vi "Resize FP.vi"(0 "VI in":refnum<vi>, 11 "error in":errorcluster) -> (4 "VI out":refnum<vi>, 15 "error out":errorcluster)   [LabVIEW 2017, in "Align To Connector.lvlib"]
uses:
  Align To Connector.lvlib
  <vilib>/Utility/miscctls.llb/LVRectTypeDef.ctl
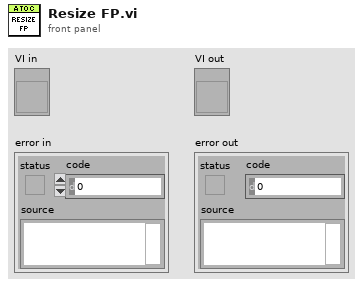
[diagram p1: front panel]
types:
  T1 = typedef "LVRectTypeDef.ctl" = cluster{"Left":i16, "Top":i16, "Right":i16, "Bottom":i16}
  T2 = typedef "LVPointTypeDef.ctl" = cluster{"Horizontal":i16, "Vertical":i16}
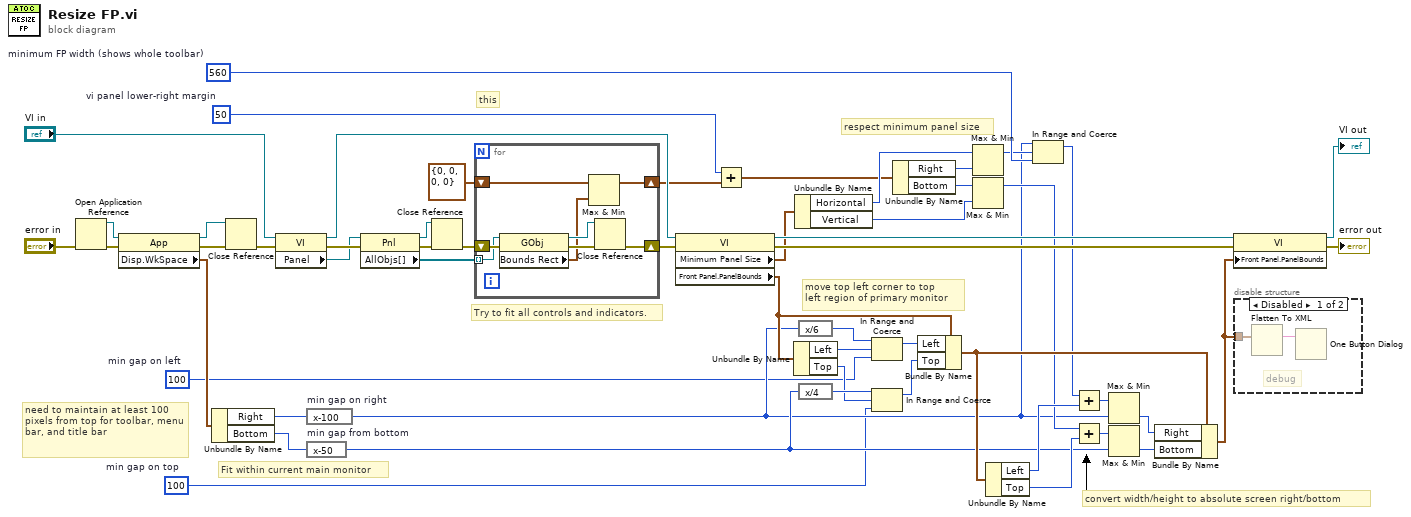
[diagram p0: block diagram]
diagram:
  w1 = i16 50  # vi panel lower-right margin
  w4 = i16 100  # min gap on left
  w7 = i16 100  # min gap on top
  w21 = i16 560  # minimum FP width (shows whole toolbar)
  # "this"
  # "respect minimum panel size"
  # "need to maintain at least 100 pixels from top for toolbar, menu bar, and title bar"
  # "move top left corner to top\nleft region of primary monitor"
  # "convert width/height to absolute screen right/bottom"
  # "Try to fit all controls and indicators."
  # "Fit within current main monitor"
  n1 = Open Application Reference(8:"error in") -> (0:w42:errorcluster, 3:w45:refnum<vi>)  [unwired: 3 in]
  n2 = property class="App"(reference=w45, error in=w42) -> (reference out=w44:refnum<vi>, error out=w43:errorcluster, "Disp.WkSpace"=w15:T1)
  n3 = Unbundle By Name(w15) -> ("Right"=w39:i16, "Bottom"=w38:i16)
  n4 = Close Reference(reference=w44, error in (no error)=w43) -> (error out=w40:errorcluster)
  n5 = property class="VI"(reference="VI in", error in=w40) -> (reference out=w30:refnum<vi>, error out=w35:errorcluster, "Panel"=w31:refnum<vi>)
  n6 = expression code="x-100" "min gap on right"(w39) -> (w10:i16)
  n7 = expression code="x-50" "min gap from bottom"(w38) -> (w20:i16)
  n8 = property class="Pnl"(reference=w31, error in=w35) -> (reference out=w33:refnum<vi>, error out=w34:errorcluster, "AllObjs[]"=w36:refnum<vi>[])
  n9 = Close Reference(reference=w33, error in (no error)=w34) -> (error out=w51:errorcluster)
  n10 = for {
    tunnel: w36 -> [w55] mode=indexing
    shift-right: [w60] -> w32
    shift-left: w51 -> [w62]
    shift-right: [w56] -> w11
    shift-left: T1 {"Left"=0, "Top"=0, "Right"=0, "Bottom"=0} ("Bounds Rect") -> [w57]
    n11 = property class="GObj"(reference=w55, error in=w62) -> (reference out=w59:refnum<vi>, error out=w61:errorcluster, "Bounds Rect"=w58:T1)
    n12 = Max & Min(x=w57, y=w58) -> (max(x,y)=w56:T1)  [unwired: 1 out]
    n13 = Close Reference(reference=w59, error in (no error)=w61) -> (error out=w60:errorcluster)
  }
  n14 = property class="VI"(reference=w30, error in=w32) -> (reference out=w52:refnum<vi>, error out=w50:errorcluster, "Minimum Panel Size"=w5:T2, "Front Panel.PanelBounds"=w16:T1)
  n15 = Add(x=w1, y=w11) -> (x+y=w2:T1)
  n16 = Unbundle By Name(w16) -> ("Left"=w53:i16, "Top"=w8:i16)
  n17 = Unbundle By Name(w5) -> ("Horizontal"=w14:i16, "Vertical"=w3:i16)
  n18 = expression code="x/6"(w10) -> (w19:i16)
  n19 = expression code="x/4"(w20) -> (w9:i16)
  n20 = In Range and Coerce(upper limit=w19, x=w53, lower limit=w4) -> (coerced(x)=w18:i16)  [unwired: 1 out]
  n21 = In Range and Coerce(upper limit=w9, x=w8, lower limit=w7) -> (coerced(x)=w17:i16)  [unwired: 1 out]
  n22 = Unbundle By Name(w2) -> ("Right"=w28:i16, "Bottom"=w27:i16)
  n23 = Bundle By Name(cluster=w16, "Left"=w18, "Top"=w17) -> (w54:T1)
  n24 = Max & Min(x=w14, y=w28) -> (max(x,y)=w13:i16)  [unwired: 1 out]
  n25 = Max & Min(x=w27, y=w3) -> (max(x,y)=w12:i16)  [unwired: 1 out]
  n26 = Unbundle By Name(w54) -> ("Left"=w46:i16, "Top"=w37:i16)
  n27 = In Range and Coerce(upper limit=w10, x=w13, lower limit=w21) -> (coerced(x)=w22:i16)  [unwired: 1 out]
  n28 = Add(x=w22, y=w46) -> (x+y=w26:i16)
  n29 = Add(x=w12, y=w37) -> (x+y=w25:i16)
  n30 = Max & Min(x=w26, y=w10) -> (min(x,y)=w24:i16)  [unwired: 1 out]
  n31 = Max & Min(x=w25, y=w20) -> (min(x,y)=w23:i16)  [unwired: 1 out]
  n32 = Bundle By Name(cluster=w54, "Right"=w24, "Bottom"=w23) -> (w6:T1)
  n33 = property class="VI"(reference=w52, error in=w50, "Front Panel.PanelBounds"=w6) -> (reference out=→"VI out":refnum<vi>, error out=→"error out":errorcluster)
  n34 = disable-structure shown="Disabled" {
    disable-tunnel: w6 -> [w64 _]
    frame Disabled {
      # "debug"
      n35 = Flatten To XML(anything=w64) -> (xml string=w63:string)
      n36 = One Button Dialog(message=w63) -> ()  [unwired: 1 in, 1 out]
    }
    frame Enabled {
    }
  }
